vi "Read Connection Type.vi"(8 "error in (no error)":errorcluster, 11 "Instrument in":refnum<class "Instrument Driver.lvclass">) -> (0 "error out":errorcluster, 2 "Connection Type":T1=enum."SwitchBlock Device", 3 "Instrument out":refnum<class "Instrument Driver.lvclass">)   [LabVIEW 2020, in "Instrument Driver.lvlib" / "Instrument Driver.lvclass"]
doc: "Read the Connection Type from the Instrument."
uses:
  Instrument Driver.lvclass
  Controls/Ctl_ConnectionType.ctl
  Instrument Driver.lvclass/Instrument Driver.ctl
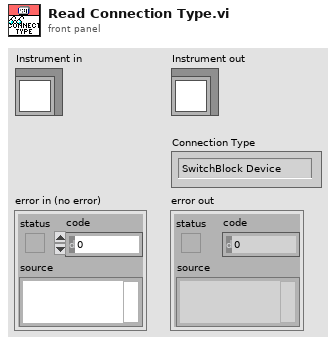
[diagram p1: front panel]
types:
  T1 = typedef "Instrument Driver.lvlib/Instrument Driver.lvclass/Ctl_ConnectionType.ctl" = enum16{"BuiltIn/System", "PXI/PCI", "USB", "GPIB", "VXI", "Serial", "TCP/IP", "cRIO", "SCXI", "cDAQ", "SwitchBlock", "SCC", "FireWire", "Accessory", "CAN", "SwitchBlock Device"}
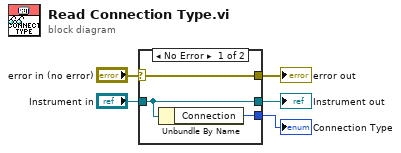
[diagram p0: block diagram]
diagram:
  n1 = case shown="No Error" "error in (no error)" {
    selector: "error in (no error)" -> [w8 w9]
    tunnel: [w8 w9] -> w4
    tunnel: [w7 w10] -> w2
    tunnel: "Instrument in" -> [w7 w10]
    tunnel: [w6 _] -> w1
    frame No Error {
      n2 = Unbundle By Name(w7) -> ("Connection"=w6:T1)
    }
    frame Error {
    }
  }
  "error out" <- w4
  "Instrument out" <- w2
  "Connection Type" <- w1
